vi "FileIO-Scan for String.vi"(0 "File Refnum":refnum<file>, 7 "regular expression":string, 11 "error IO":errorcluster) -> (4 "refnum out":refnum<file>, 6 "lines before match":string[](array[string]), 8 "matched line":string, 15 "error out":errorcluster)   [LabVIEW 2020]
panel:
  out "Numeric":i32
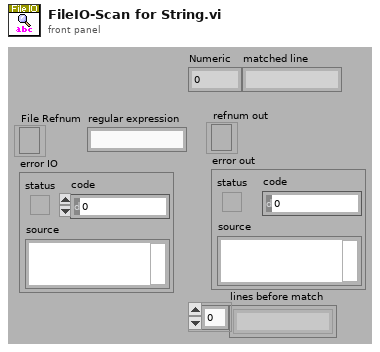
[diagram p1: front panel]
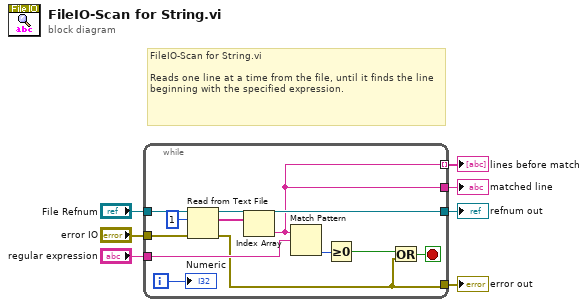
[diagram p0: block diagram]
diagram:
  # "FileIO-Scan for String.vi\n\nReads one line at a time from the file, until it finds the line beginning with the specified expression."
  n1 = while {
    tunnel: "error IO" -> [w19]
    tunnel: "File Refnum" -> [w18]
    tunnel: [w8] -> w3
    tunnel: [w15] -> w4
    tunnel: "regular expression" -> [w12]
    tunnel: [w9] -> w2
    tunnel: [w9] -> w1 mode=indexing
    i -> [w11]
    stop <- w14 stop-if-true
    n2 = Read from Text File(file (use dialog)=w18, count=1, error in=w19) -> (refnum out=w15:refnum<file>, text=w10:string[], error out=w8:errorcluster)  [unwired: 1 in, 1 out]
    n3 = Index Array(array=w10) -> (element=w9:string)  [unwired: 1 in]
    n4 = Match Pattern(string=w9, regular expression=w12) -> (offset past match=w16:i32)  [unwired: 1 in, 3 out]
    n5 = Greater Or Equal To 0?(x=w16) -> (x >= 0?=w13:bool)
    n6 = Or(x=w13, y=w8) -> (x .or. y?=w14:bool)
    "Numeric" <- w11
  }
  "refnum out" <- w4
  "error out" <- w3
  "matched line" <- w2
  "lines before match" <- w1
